vi "Get Variables.vi"(8 "error in (no error)":errorcluster, 11 "Message Popup in":refnum<class "Message Popup.lvclass">) -> (0 "error out":errorcluster, 2 "Variables":variant, 3 "Message Popup out":refnum<class "Message Popup.lvclass">)   [LabVIEW 2016, in "Message Popup.lvclass"]
uses:
  Message Popup.lvclass
  Variables.ctl
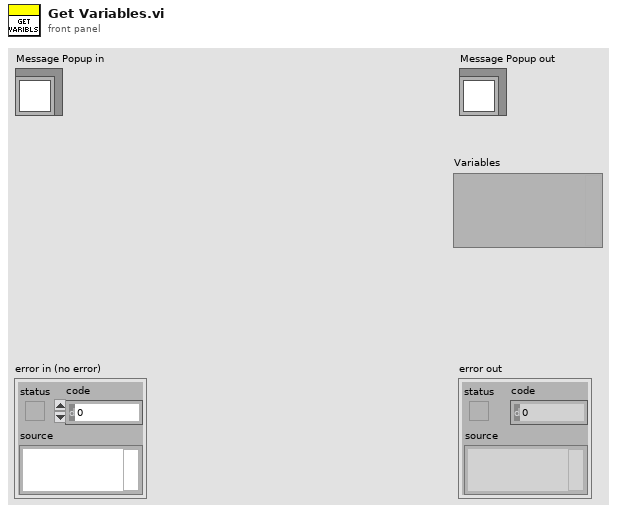
[diagram p1: front panel]
types:
  T1 = typedef "Message Popup.lvclass/Variables.ctl" = cluster{"Message":string}
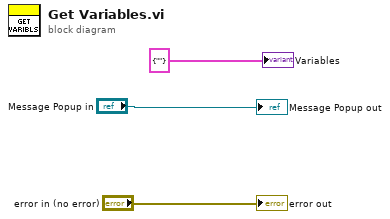
[diagram p0: block diagram]
diagram:
  "error out" <- "error in (no error)"
  "Message Popup out" <- "Message Popup in"
  "Variables" <- T1 {"Message"=""} ("Variables")
